vi "运维调试界面.vi"() -> ()   [LabVIEW 2016, in "质控单元V4.lvlib"]
uses:
  <vilib>/Utility/miscctls.llb/LVPointTypeDef.ctl
  <vilib>/ptbypt/NI_PtbyPt.lvlib
panel:
  out "权限等级":string
  in  "布尔":bool
  in  "ZK定时设置":cluster{"启动":bool, "控制命令":T1, "测量参数":T2}(xcontrol)
  out "模块版本号":string
  in  "Tab Control 7":enum32{"参数"}(tab)
  out "CODMn运行模式":string caption="运行模式"
  out "CODmn运行流程":string caption="运行状态"
  in  "CODMn启用":bool caption="启用"
  out "CODMn剩余时间":string caption="剩余时间"
  out "CODMn当前步骤":string caption="当前步骤"
  out "CODMn当前流程":string caption="当前流程"
  out "CODMn告警状态":string caption="告警状态"
  out "CODMn液位状态":string caption="液位状态"
  out "CODMn运行状态":string caption="质控状态"
  out "CODMn通讯状态":bool caption="状态"
  in  "Tab Control 6":enum32{"参数"}(tab)
  out "总氮运行模式":string caption="运行模式"
  out "总氮运行流程":string caption="运行状态"
  in  "总氮启用":bool caption="启用"
  out "TN剩余时间":string caption="剩余时间"
  out "TN当前步骤":string caption="当前步骤"
  out "TN当前流程":string caption="当前流程"
  out "TN告警状态":string caption="告警状态"
  out "TN液位状态":string caption="液位状态"
  out "TN运行状态":string caption="质控状态"
  out "TN通讯状态":bool caption="状态"
  in  "Tab Control 5":enum32{"参数"}(tab)
  out "总磷运行模式":string caption="运行模式"
  out "总磷运行流程":string caption="运行状态"
  in  "总磷启用":bool caption="启用"
  out "TP剩余时间":string caption="剩余时间"
  out "TP当前步骤":string caption="当前步骤"
  out "TP当前流程":string caption="当前流程"
  out "TP告警状态":string caption="告警状态"
  out "TP液位状态":string caption="液位状态"
  out "TP运行状态":string caption="质控状态"
  out "TP通讯状态":bool caption="状态"
  in  "Tab Control 4":enum32{"参数"}(tab)
  out "氨氮运行模式":string caption="运行模式"
  out "氨氮剩余时间":string caption="剩余时间"
  out "氨氮当前步骤":string caption="当前步骤"
  out "氨氮当前流程":string caption="当前流程"
  out "氨氮告警状态":string caption="告警状态"
  out "氨氮液位状态":string caption="液位状态"
  out "氨氮运行状态":string caption="质控状态"
  out "氨氮通讯状态":bool caption="状态"
  in  "氨氮启用":bool caption="启用"
  out "氨氮运行流程":string caption="运行状态"
  in  "停止":bool
  in  "参数设置":bool
  in  "连接设置":bool
  in  "调试界面":bool
  in  "加标回收":bool
  # "CODMn质控状态"
  # "总氮质控状态"
  # "总磷质控状态"
  # "氨氮质控状态"
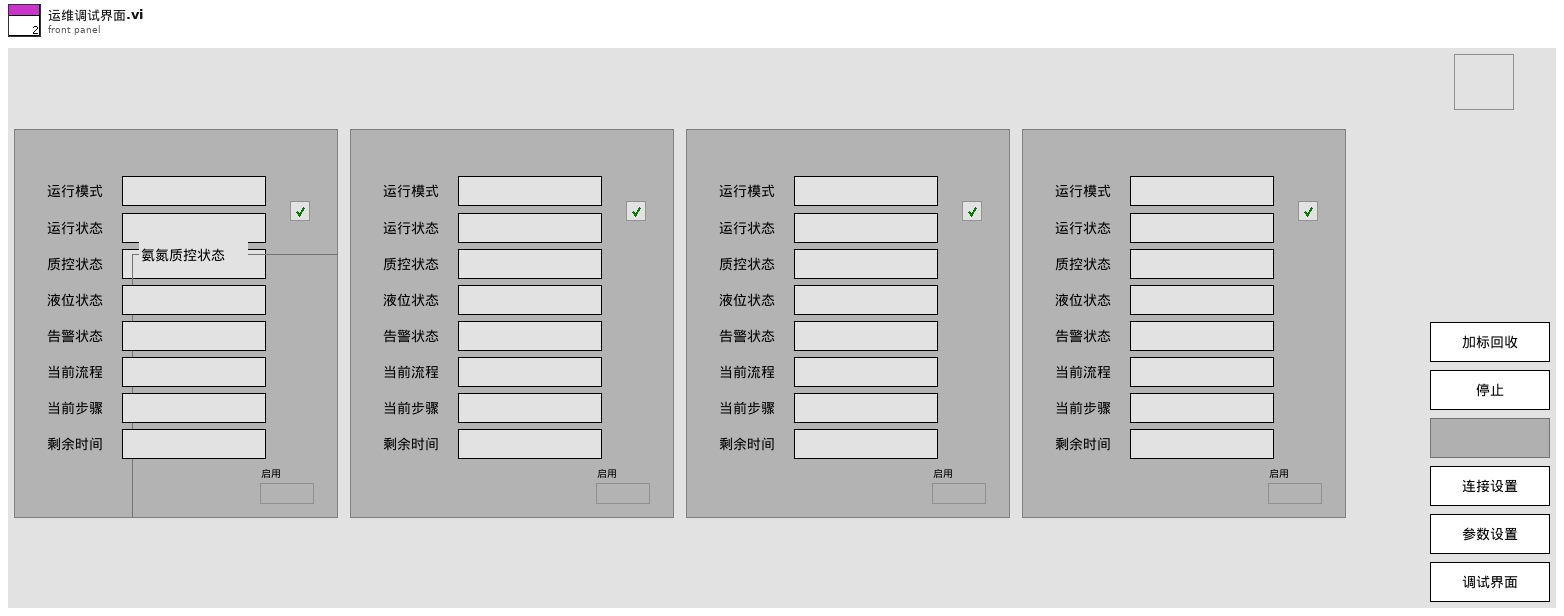
[diagram p1: front panel]
types:
  T1 = typedef "ZK定时设置.xctl/国标控制命令.ctl" = enum16{"加标回收（启动采配水）", "加标回收（不启动采配水）", "水样测试（启动采配水）", "水样测试（不启动采配水）"}
  T2 = typedef "ZK定时设置.xctl/测量参数.ctl" = cluster{"氨氮":bool, "总磷":bool, "总氮":bool, "CODMn":bool, "CODCr":bool}
  T3 = typedef "质控单元V4.lvlib/数据流类型.ctl" = cluster{"cmd":enum16{"start", "stop"}, "data":variant}
  T4 = typedef "LVPointTypeDef.ctl" = cluster{"Horizontal":i16, "Vertical":i16}
  T5 = cluster{"启用参数选择":cluster{"氨氮启用":bool, "总磷启用":bool, "总氮启用":bool, "CODMn启用":bool, "CODCr启用":bool}, "流程":enum16{"加标回收（启动采配水）", "加标回收（不启动采配水）", "水样测试（启动采配水）", "水样测试（不启动采配水）"}}
  T6 = cluster{"氨氮启用":bool, "总磷启用":bool, "总氮启用":bool, "CODMn启用":bool, "CODCr启用":bool}
  T7 = enum16{"加标回收（启动采配水）", "加标回收（不启动采配水）", "水样测试（启动采配水）", "水样测试（不启动采配水）"}
  T8 = cluster{"氨氮":bool, "总磷":bool, "总氮":bool, "CODMn":bool, "CODCr":bool, "氨氮总磷":bool, "总磷总氮":bool}
  T9 = cluster{"启动参数":cluster{"氨氮启用":bool, "总磷启用":bool, "总氮启用":bool, "CODMn启用":bool, "CODCr启用":bool}, "流程参数":enum16{"加标回收（启动采配水）", "加标回收（不启动采配水）", "水样测试（启动采配水）", "水样测试（不启动采配水）"}}
  T10 = typedef "质控单元V4.lvlib/质控仪器状态显示.ctl" = cluster{"运行模式":string, "运行状态":string, "液位状态":string, "告警状态":string, "当前流程":string, "当前步骤":string, "剩余时间":string}
  T11 = cluster{"Major":u16, "Minor":u16, "Fix":u16, "Build":u16}
  T12 = enum8{"Enabled", "Disabled", "Disabled and Grayed Out"}
  T13 = cluster{"氨氮":bool, "总磷":bool, "总氮":bool, "CODMn":bool, "CODCr":bool}
  T14 = enum32{"Bad", "Idle", "Run top level", "Running"}
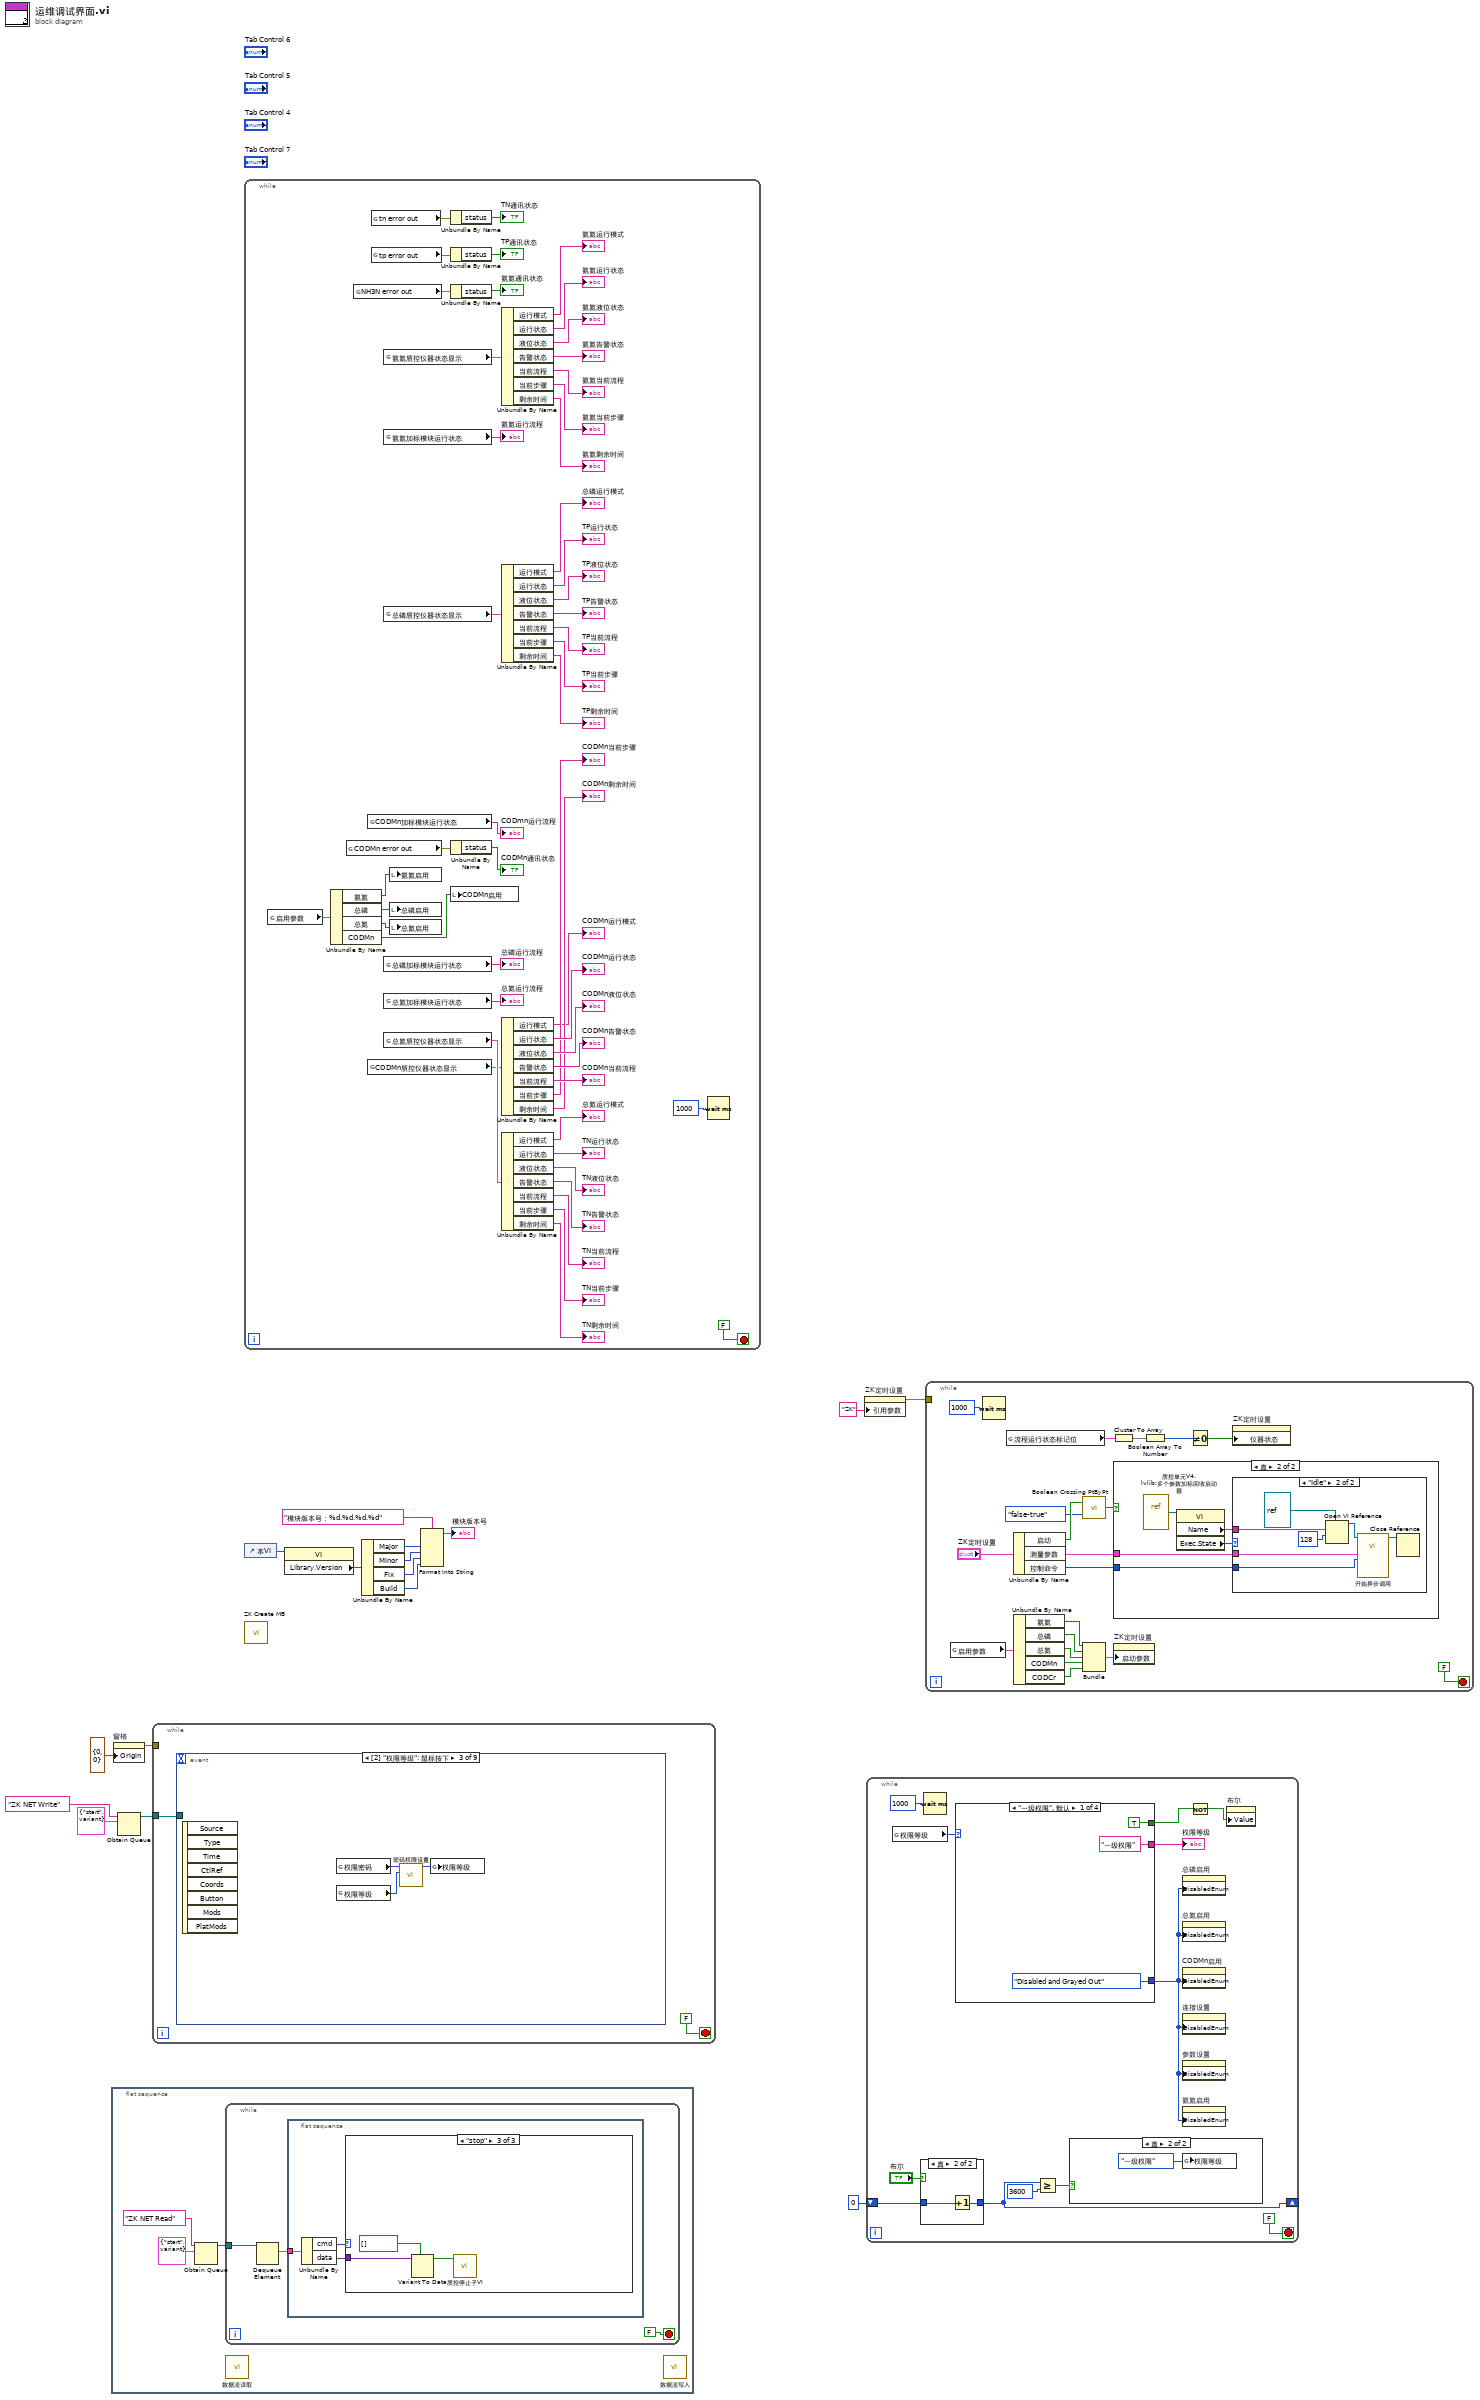
[diagram p0: block diagram]
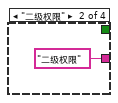
[diagram p2: hidden frame]
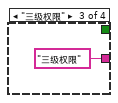
[diagram p3: hidden frame]
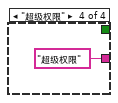
[diagram p4: hidden frame]
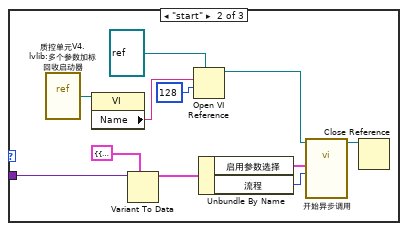
[diagram p8: hidden frame]
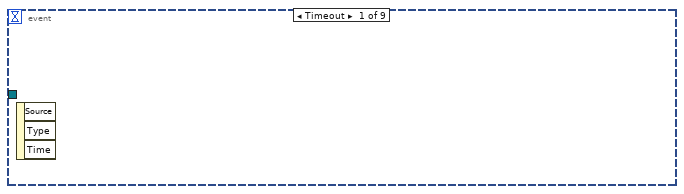
[diagram p11: hidden frame]
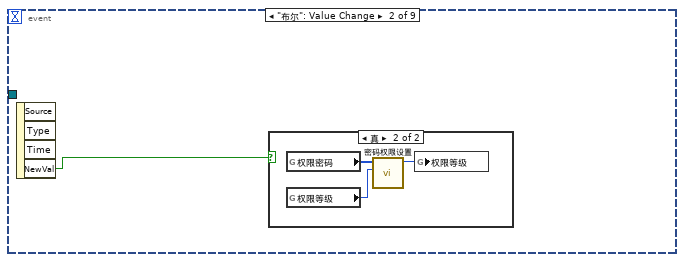
[diagram p12: hidden frame]
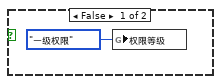
[diagram p13: hidden frame]
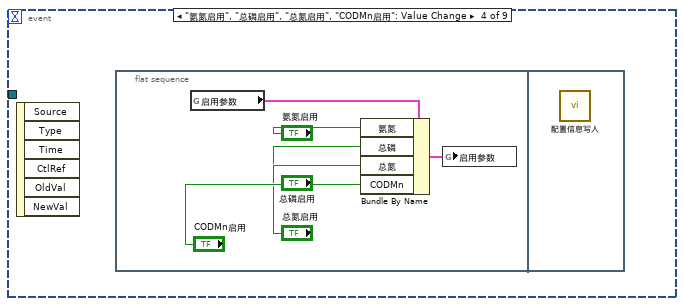
[diagram p14: hidden frame]
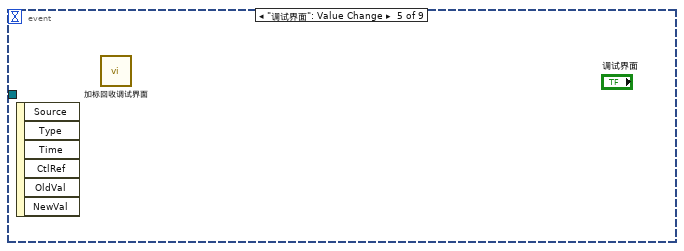
[diagram p15: hidden frame]
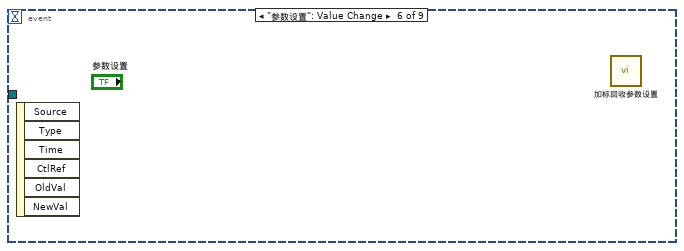
[diagram p16: hidden frame]
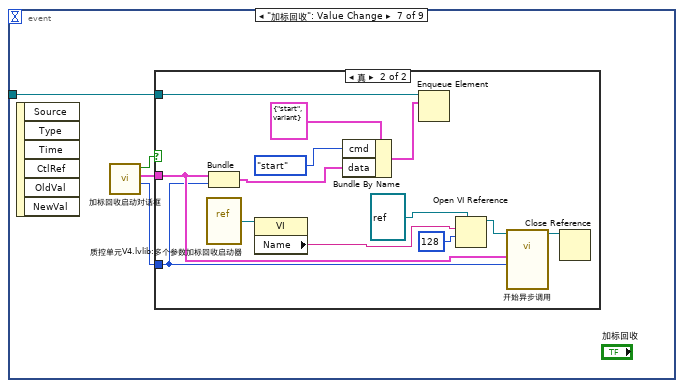
[diagram p17: hidden frame]
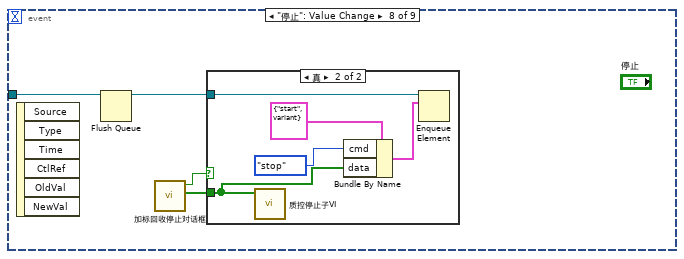
[diagram p19: hidden frame]
diagram:
  n1 = flat-sequence {
    frame #0 {
      n2 = Obtain Queue(name (unnamed)="ZK NET Read" ("名称（未命名）"), element data type=T3 {"cmd"=enum."start", "data"=variant} ("簇")) -> (queue out=w18:refnum<queue>)  [unwired: 3 in, 2 out]
      n3 = while {
        tunnel: w18 -> [w22]
        stop <- FALSE stop-if-true
        n4 = Dequeue Element(queue=w22) -> (element=w20:T3)  [unwired: 2 in, 3 out]
        n5 = flat-sequence {
          tunnel: w20 -> [w25]
          frame #0 {
            n6 = Unbundle By Name(w25) -> ("cmd"=w24:enum16{"start", "stop"}, "data"=w23:variant)
            n7 = case shown="\"stop\"" w24 {
              tunnel: w23 -> [_ w30 w39]
              frame Default {
              }
              frame "start" {
                n8 = vi-ref "质控单元V4.lvlib:多个参数加标回收启动器.vi"() -> (w36:refnum<vi>)
                n9 = property class="VI"(reference=w36) -> ("Name"=w35:string)  [unwired: 1 in, 2 out]
                n10 = Variant To Data(type=T5 {"启用参数选择"={"氨氮启用"=FALSE, "总磷启用"=FALSE, "总氮启用"=FALSE, "CODMn启用"=FALSE, "CODCr启用"=FALSE}, "流程"=enum."加标回收（启动采配水）"} ("data"), Variant=w30) -> (data=w28:T5)  [unwired: 1 in, 1 out]
                n11 = Open VI Reference(type specifier VI Refnum (for type only)=refnum<vi> refnum, vi path=w35, options=128 ("选项")) -> (vi reference=w33:refnum<vi>)  [unwired: 3 in, 1 out]
                n12 = Unbundle By Name(w28) -> ("启用参数选择"=w27:T6, "流程"=w26:T7)
                n13 = call-by-ref "开始异步调用"(reference=w33, "流程"=w26, "启用参数选择"=w27) -> (reference out=w32:refnum<vi>)  [unwired: 11 in, 1 out]
                n14 = Close Reference(reference=w32) -> ()  [unwired: 1 in, 1 out]
              }
              frame "stop" {
                n15 = Variant To Data(type=bool[] [] ("数组"), Variant=w39) -> (data=w37:bool[])  [unwired: 1 in, 1 out]
                n16 = call "质控停止子VI.vi"("数组"=w37) -> ()  [unwired: 11 in]
              }
            }
          }
        }
      }
      n17 = call "数据流读取.vi"() -> ()  [unwired: 12 in]
      n18 = call "数据流写入.vi"() -> ()  [unwired: 12 in]
    }
  }
  n19 = property on="窗格" class="Pane"("Origin"=T4 {"Horizontal"=0, "Vertical"=0} ("原点")) -> (error out=w15:errorcluster)  [unwired: 2 in, 1 out]
  n20 = Obtain Queue(name (unnamed)="ZK NET Write" ("名称（未命名）"), element data type=T3 {"cmd"=enum."start", "data"=variant} ("簇")) -> (queue out=w3:refnum<queue>)  [unwired: 3 in, 2 out]
  n21 = while {
    tunnel: w15 -> [_]
    tunnel: w3 -> [w40]
    stop <- FALSE stop-if-true
    n22 = event shown="[2] \"权限等级\": 鼠标按下" {
      selector: _ -> [_ _ _ _ _ _ _ _ _]
      dyn-events: _ -> [_ _ _ _ _ _ _ _ _]
      timeout: _ -> [_ _ _ _ _ _ _ _ _]
      tunnel: w40 -> [_ _ _ _ _ _ w56 w76 _]
      event Timeout {
        n23 = event-data() -> ()  [unwired: 1 in, 3 out]
      }
      event "布尔": Value Change {
        n24 = event-data() -> ("NewVal"=w42:bool)  [unwired: 1 in, 3 out]
        n25 = case shown="真" w42 {
          frame False {
            n26 = global write "ZK非断电保存全局变量.vi" "权限等级"(enum16{"一级权限", "二级权限", "三级权限", "超级权限"}."一级权限" ("权限等级")) -> ()
          }
          frame True {
            n27 = global read "ZK非断电保存全局变量.vi" "权限密码"() -> (w46:u32[])
            n28 = global read "ZK非断电保存全局变量.vi" "权限等级"() -> (w44:enum16{"一级权限", "二级权限", "三级权限", "超级权限"})
            n29 = call "密码权限设置.vi"("权限输入"=w44, "权限密码"=w46) -> ("权限输出"=w45:enum16{"一级权限", "二级权限", "三级权限", "超级权限"})  [unwired: 9 in]
            n30 = global write "ZK非断电保存全局变量.vi" "权限等级"(w45) -> ()
          }
        }
      }
      event "权限等级": Mouse Down {
        n31 = event-data() -> ()  [unwired: 1 in, 8 out]
        n32 = global read "ZK非断电保存全局变量.vi" "权限密码"() -> (w49:u32[])
        n33 = global read "ZK非断电保存全局变量.vi" "权限等级"() -> (w47:enum16{"一级权限", "二级权限", "三级权限", "超级权限"})
        n34 = call "密码权限设置.vi"("权限输入"=w47, "权限密码"=w49) -> ("权限输出"=w48:enum16{"一级权限", "二级权限", "三级权限", "超级权限"})  [unwired: 9 in]
        n35 = global write "ZK非断电保存全局变量.vi" "权限等级"(w48) -> ()
      }
      event "氨氮启用", "总磷启用", "总氮启用", "CODMn启用": Value Change {
        n36 = event-data() -> ()  [unwired: 1 in, 6 out]
        n37 = flat-sequence {
          frame #0 {
            n38 = global read "ZK断电保存全局变量.vi" "启用参数"() -> (w50:T8)
            n39 = Bundle By Name(cluster=w50, "氨氮"="氨氮启用", "总磷"="总磷启用", "总氮"="总氮启用", "CODMn"="CODMn启用") -> (w51:T8)
            n40 = global write "ZK断电保存全局变量.vi" "启用参数"(w51) -> ()
          }
          frame #1 {
            n41 = call "配置信息写入.vi"() -> ()  [unwired: 11 in, 1 out]
          }
        }
      }
      event "调试界面": Value Change {
        n42 = event-data() -> ()  [unwired: 1 in, 6 out]
        n43 = call "加标回收调试界面.vi"() -> ()  [unwired: 12 in]
      }
      event "参数设置": Value Change {
        n44 = event-data() -> ()  [unwired: 1 in, 6 out]
        n45 = call "加标回收参数设置.vi"() -> ()  [unwired: 12 in]
      }
      event "加标回收": Value Change {
        n46 = event-data() -> ()  [unwired: 1 in, 6 out]
        n47 = call "加标回收启动对话框.vi"() -> ("流程参数"=w57:T7, "启动参数"=w58:T6, "check ？"=w59:bool)  [unwired: 9 in]
        n48 = case shown="真" w59 {
          tunnel: w58 -> [_ w65]
          tunnel: w57 -> [_ w64]
          tunnel: w56 -> [_ w66]
          frame False {
          }
          frame True {
            n49 = vi-ref "质控单元V4.lvlib:多个参数加标回收启动器.vi"() -> (w72:refnum<vi>)
            n50 = Bundle("启动参数"=w65, "流程参数"=w64) -> (w61:T9)  [unwired: 1 in]
            n51 = property class="VI"(reference=w72) -> ("Name"=w71:string)  [unwired: 1 in, 2 out]
            n52 = Bundle By Name(cluster=T3 {"cmd"=enum."start", "data"=variant} ("簇"), "cmd"=enum16{"start", "stop"}."start", "data"=w61) -> (w60:T3)
            n53 = Enqueue Element(queue=w66, element=w60) -> ()  [unwired: 2 in, 3 out]
            n54 = Open VI Reference(type specifier VI Refnum (for type only)=refnum<vi> refnum, vi path=w71, options=128 ("选项")) -> (vi reference=w69:refnum<vi>)  [unwired: 3 in, 1 out]
            n55 = call-by-ref "开始异步调用"(reference=w69, "流程"=w64, "启用参数选择"=w65) -> (reference out=w68:refnum<vi>)  [unwired: 11 in, 1 out]
            n56 = Close Reference(reference=w68) -> ()  [unwired: 1 in, 1 out]
          }
        }
      }
      event "停止": Value Change {
        n57 = event-data() -> ()  [unwired: 1 in, 6 out]
        n58 = Flush Queue(queue=w76) -> (queue out=w75:refnum<queue>)  [unwired: 1 in, 2 out]
        n59 = call "加标回收停止对话框.vi"() -> ("数组"=w74:bool[], "check？"=w73:bool)  [unwired: 10 in]
        n60 = case shown="真" w73 {
          tunnel: w75 -> [_ w81]
          tunnel: w74 -> [_ w77]
          frame False {
          }
          frame True {
            n61 = call "质控停止子VI.vi"("数组"=w77) -> ()  [unwired: 11 in]
            n62 = Bundle By Name(cluster=T3 {"cmd"=enum."start", "data"=variant} ("簇"), "cmd"=enum16{"start", "stop"}."stop", "data"=w77) -> (w78:T3)
            n63 = Enqueue Element(queue=w81, element=w78) -> ()  [unwired: 2 in, 3 out]
          }
        }
      }
      event "连接设置": Value Change {
        n64 = event-data() -> ()  [unwired: 1 in, 6 out]
        n65 = call "串口配置.vi"() -> ()  [unwired: 12 in]
      }
    }
  }
  n66 = while {
    stop <- FALSE stop-if-true
    n67 = global read "ZK断电保存全局变量.vi" "启用参数"() -> (w90:T8)
    n68 = Unbundle By Name(w90) -> ("氨氮"=w89:bool, "总磷"=w88:bool, "总氮"=w87:bool, "CODMn"=w86:bool)
    n69 = global read "ZK非断电保存全局变量.vi" "CODMn error out"() -> (w130:errorcluster)
    n70 = global read "ZK非断电保存全局变量.vi" "NH3N error out"() -> (w129:errorcluster)
    n71 = global read "ZK非断电保存全局变量.vi" "CODMn加标模块运行状态"() -> (→"CODmn运行流程":string)
    n72 = global read "ZK非断电保存全局变量.vi" "CODMn质控仪器状态显示"() -> (w106:T10)
    n73 = global read "ZK非断电保存全局变量.vi" "tn error out"() -> (w97:errorcluster)
    n74 = global read "ZK非断电保存全局变量.vi" "tp error out"() -> (w98:errorcluster)
    n75 = global read "ZK非断电保存全局变量.vi" "氨氮质控仪器状态显示"() -> (w127:T10)
    n76 = global read "ZK非断电保存全局变量.vi" "氨氮加标模块运行状态"() -> (→"氨氮运行流程":string)
    n77 = global read "ZK非断电保存全局变量.vi" "总磷质控仪器状态显示"() -> (w120:T10)
    n78 = global read "ZK非断电保存全局变量.vi" "总磷加标模块运行状态"() -> (→"总磷运行流程":string)
    n79 = global read "ZK非断电保存全局变量.vi" "总氮加标模块运行状态"() -> (→"总氮运行流程":string)
    n80 = global read "ZK非断电保存全局变量.vi" "总氮质控仪器状态显示"() -> (w113:T10)
    n81 = local write "氨氮启用"(w89) -> ()
    n82 = local write "总磷启用"(w88) -> ()
    n83 = local write "总氮启用"(w87) -> ()
    n84 = Unbundle By Name(w97) -> ("status"=→"TN通讯状态":bool)
    n85 = Unbundle By Name(w98) -> ("status"=→"TP通讯状态":bool)
    n86 = Unbundle By Name(w129) -> ("status"=→"氨氮通讯状态":bool)
    n87 = Unbundle By Name(w130) -> ("status"=→"CODMn通讯状态":bool)
    n88 = local write "CODMn启用"(w86) -> ()
    n89 = Unbundle By Name(w127) -> ("运行模式"=→"氨氮运行模式":string, "运行状态"=→"氨氮运行状态":string, "液位状态"=→"氨氮液位状态":string, "告警状态"=→"氨氮告警状态":string, "当前流程"=→"氨氮当前流程":string, "当前步骤"=→"氨氮当前步骤":string, "剩余时间"=→"氨氮剩余时间":string)
    n90 = Unbundle By Name(w120) -> ("运行模式"=→"总磷运行模式":string, "运行状态"=→"TP运行状态":string, "液位状态"=→"TP液位状态":string, "告警状态"=→"TP告警状态":string, "当前流程"=→"TP当前流程":string, "当前步骤"=→"TP当前步骤":string, "剩余时间"=→"TP剩余时间":string)
    n91 = Unbundle By Name(w106) -> ("运行模式"=→"CODMn运行模式":string, "运行状态"=→"CODMn运行状态":string, "液位状态"=→"CODMn液位状态":string, "告警状态"=→"CODMn告警状态":string, "当前流程"=→"CODMn当前流程":string, "当前步骤"=→"CODMn当前步骤":string, "剩余时间"=→"CODMn剩余时间":string)
    n92 = Unbundle By Name(w113) -> ("运行模式"=→"总氮运行模式":string, "运行状态"=→"TN运行状态":string, "液位状态"=→"TN液位状态":string, "告警状态"=→"TN告警状态":string, "当前流程"=→"TN当前流程":string, "当前步骤"=→"TN当前步骤":string, "剩余时间"=→"TN剩余时间":string)
    n93 = Wait (ms)(milliseconds to wait=u32 1000 ("等待时间（毫秒）")) -> ()  [unwired: 1 out]
  }
  n94 = control-ref of="本VI"() -> (w14:refnum<vi>)
  n95 = call "ZK Create MB.vi"() -> ()  [unwired: 12 in]
  n96 = property class="VI"(reference=w14) -> ("Library.Version"=w13:T11)  [unwired: 1 in, 2 out]
  n97 = Unbundle By Name(w13) -> ("Major"=w11:u16, "Minor"=w10:u16, "Fix"=w9:u16, "Build"=w8:u16)
  n98 = Format Into String(format string="模块版本号：%d.%d.%d.%d" ("格式字符串"), w11, w10, w9, w8) -> (resulting string=→"模块版本号":string)  [unwired: 2 in, 1 out]
  n99 = property on="ZK定时设置" class="ZK定时设置 (严格)"("引用参数"="ZK") -> (error out=w5:errorcluster)  [unwired: 2 in, 1 out]
  n100 = while {
    shift-right: [w143] -> _
    shift-left: 0 -> [w144]
    stop <- FALSE stop-if-true
    n101 = global read "ZK非断电保存全局变量.vi" "权限等级"() -> (w138:enum16{"一级权限", "二级权限", "三级权限", "超级权限"})
    n102 = case shown="真" "布尔" {
      tunnel: w144 -> [_ w153]
      tunnel: [_ w152] -> w143
      frame False {
      }
      frame True {
        n103 = Increment(x=w153) -> (x+1=w152:i32)
      }
    }
    n104 = Wait (ms)(milliseconds to wait=u32 1000 ("等待时间（毫秒）")) -> ()  [unwired: 1 out]
    n105 = case shown="\"一级权限\", 默认" w138 {
      tunnel: [T12."Disabled and Grayed Out" ("禁用") _ _ _] -> w137
      tunnel: ["一级权限" "二级权限" "三级权限" "超级权限"] -> w135
      tunnel: [TRUE ("布尔") _ _ _] -> w134
      frame "一级权限", Default {
      }
      frame "二级权限" {
      }
      frame "三级权限" {
      }
      frame "超级权限" {
      }
    }
    "权限等级" <- w135
    n106 = Greater Or Equal?(x=w143, y=3600) -> (x >= y?=w141:bool)
    n107 = case shown="真" w141 {
      frame False {
      }
      frame True {
        n108 = global write "ZK非断电保存全局变量.vi" "权限等级"(enum16{"一级权限", "二级权限", "三级权限", "超级权限"}."一级权限" ("权限等级")) -> ()
      }
    }
    n109 = property on="总磷启用" class="Bool (严格)"("DisabledEnum"=w137) -> ()  [unwired: 2 in, 2 out]
    n110 = property on="总氮启用" class="Bool (严格)"("DisabledEnum"=w137) -> ()  [unwired: 2 in, 2 out]
    n111 = property on="CODMn启用" class="Bool (严格)"("DisabledEnum"=w137) -> ()  [unwired: 2 in, 2 out]
    n112 = property on="连接设置" class="Bool"("DisabledEnum"=w137) -> ()  [unwired: 2 in, 2 out]
    n113 = property on="参数设置" class="Bool"("DisabledEnum"=w137) -> ()  [unwired: 2 in, 2 out]
    n114 = property on="氨氮启用" class="Bool (严格)"("DisabledEnum"=w137) -> ()  [unwired: 2 in, 2 out]
    n115 = Not(x=w134) -> (.not. x?=w133:bool)
    n116 = property on="布尔" class="Bool (严格)"("Value"=w133) -> ()  [unwired: 2 in, 2 out]
  }
  n117 = while {
    tunnel: w5 -> [_]
    stop <- FALSE stop-if-true
    n118 = global read "ZK断电保存全局变量.vi" "启用参数"() -> (w160:T8)
    n119 = Wait (ms)(milliseconds to wait=u32 1000 ("等待时间（毫秒）")) -> ()  [unwired: 1 out]
    n120 = global read "ZK非断电保存全局变量.vi" "流程运行状态标记位"() -> (w167:T8)
    n121 = Unbundle By Name("ZK定时设置") -> ("启动"=w163:bool, "测量参数"=w169:T2, "控制命令"=w168:T1)
    n122 = Unbundle By Name(w160) -> ("氨氮"=w159:bool, "总磷"=w158:bool, "总氮"=w157:bool, "CODMn"=w156:bool, "CODCr"=w155:bool)
    n123 = call <vilib>:"Boolean Crossing PtByPt.vi"("direction"=enum16{"either", "false-true", "true-false"}."false-true", "input"=w163) -> ("crossing"=w162:bool)  [unwired: 1 in]
    n124 = Bundle("氨氮"=w159, "总磷"=w158, "总氮"=w157, "CODMn"=w156, "CODCr"=w155) -> (w154:T13)  [unwired: 1 in]
    n125 = Cluster To Array(cluster=w167) -> (array=w166:bool[])
    n126 = case shown="真" w162 {
      tunnel: w169 -> [_ w175]
      tunnel: w168 -> [_ w174]
      frame False {
      }
      frame True {
        n127 = vi-ref "质控单元V4.lvlib:多个参数加标回收启动器.vi"() -> (w176:refnum<vi>)
        n128 = property class="VI"(reference=w176) -> ("Name"=w177:string, "Exec.State"=w173:T14)  [unwired: 1 in, 2 out]
        n129 = case shown="\"Idle\"" w173 {
          tunnel: w177 -> [_ w180]
          tunnel: w175 -> [_ w179]
          tunnel: w174 -> [_ w178]
          frame "Bad", Default {
          }
          frame "Idle" {
            n130 = Open VI Reference(type specifier VI Refnum (for type only)=refnum<vi> refnum, vi path=w180, options=128 ("选项")) -> (vi reference=w182:refnum<vi>)  [unwired: 3 in, 1 out]
            n131 = call-by-ref "开始异步调用"(reference=w182, "流程"=w178, "启用参数选择"=w179) -> (reference out=w183:refnum<vi>)  [unwired: 11 in, 1 out]
            n132 = Close Reference(reference=w183) -> ()  [unwired: 1 in, 1 out]
          }
        }
      }
    }
    n133 = property on="ZK定时设置" class="ZK定时设置 (严格)"("启动参数"=w154) -> ()  [unwired: 2 in, 2 out]
    n134 = Boolean Array To Number(Boolean array=w166) -> (number=w165:u32)
    n135 = Not Equal To 0?(x=w165) -> (x != 0?=w164:bool)
    n136 = property on="ZK定时设置" class="ZK定时设置 (严格)"("仪器状态"=w164) -> ()  [unwired: 2 in, 2 out]
  }
